vi "Pre-processing (White lines on ramp).vi"(6 "error in":errorcluster, 9 "Image In":T1) -> (0 "error out":errorcluster, 2 "Number of Particles":i32, 3 "Image Out":T1)   [LabVIEW 2009]
uses:
  <vilib>/vision/Image Controls.llb/IMAQ Image.ctl
  <vilib>/vision/NI_Vision_Development_Module.lvlib
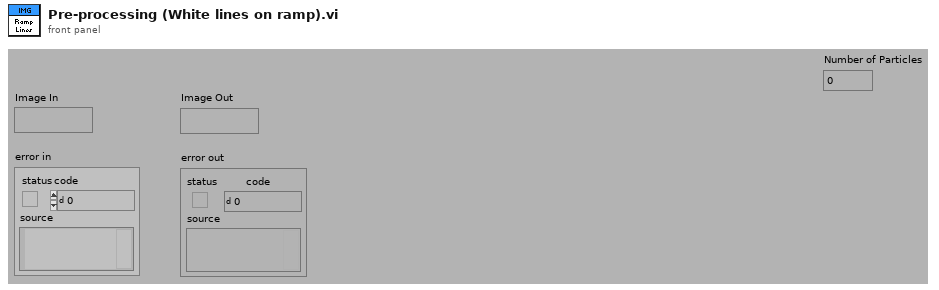
[diagram p1: front panel]
types:
  T1 = typedef "IMAQ Image.ctl" = refnum<image>
  T2 = cluster{"Measurement Parameter":i32, "Range Lower Value":dbl, "Range Upper Value":dbl, "Range":bool, "Measurement Type":bool}[]
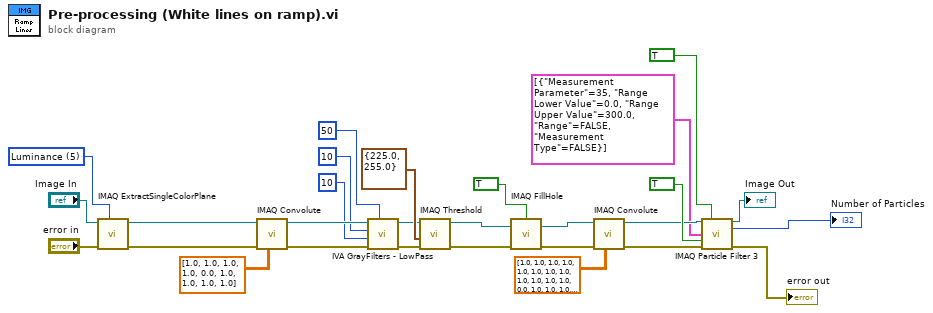
[diagram p0: block diagram]
diagram:
  w28 = 5 items=["Red", "Green", "Blue", "Hue", "Saturation", "Luminance", "Value", "Intensity"] ("Color Plane")
  n1 = call "IMAQ ExtractSingleColorPlane"("Color Plane"=w28, "error in (no error)"="error in", "Image Src"="Image In") -> ("error out"=w25:errorcluster, "Image Dst Out"=w23:T1)  [unwired: 1 in, 6 out]
  n2 = call "IMAQ Convolute"("Kernel"=sgl[][] [[1.0, 1.0, 1.0], [1.0, 0.0, 1.0], [1.0, 1.0, 1.0]], "error in (no error)"=w25, "Image Src"=w23) -> ("error out"=w22:errorcluster, "Image Dst Out"=w21:T1)  [unwired: 4 in, 3 out]
  n3 = call <vilib>:"IVA GrayFilters - LowPass.vi"("Tolerance"=50, "error in"=w22, "Filter size Y"=10, "Filter size X"=10, "Image In"=w21) -> ("error out"=w20:errorcluster, "Image Out"=w15:T1)  [unwired: 5 out]
  n4 = call "IMAQ Threshold"("error in (no error)"=w20, "Range"=cluster{"Lower value":sgl, "Upper value":sgl} {"Lower value"=225.0, "Upper value"=255.0}, "Image Src"=w15) -> ("error out"=w14:errorcluster, "Image Dst Out"=w12:T1)  [unwired: 3 in, 4 out]
  n5 = call "IMAQ FillHole"("error in (no error)"=w14, "Image Src"=w12, "Connectivity 4/8 (8)"=TRUE) -> ("error out"=w11:errorcluster, "Image Dst Out"=w9:T1)  [unwired: 1 in, 2 out]
  n6 = call "IMAQ Convolute"("Kernel"=sgl[][] [[1.0, 1.0, 1.0, 1.0, 1.0], [1.0, 1.0, 1.0, 1.0, 1.0], [1.0, 1.0, 0.0, 1.0, 1.0], [1.0, 1.0, 1.0, 1.0, 1.0], [1.0, 1.0, 1.0, 1.0, 1.0]], "error in (no error)"=w11, "Image Src"=w9) -> ("error out"=w8:errorcluster, "Image Dst Out"=w3:T1)  [unwired: 4 in, 3 out]
  n7 = call "IMAQ Particle Filter 3"("Image Src"=w3, "Connectivity 4/8 (8)"=TRUE, "Selection Values"=T2 [{"Measurement Parameter"=35, "Range Lower Value"=0.0, "Range Upper Value"=300.0, "Range"=FALSE, "Measurement Type"=FALSE}], "Keep/Remove Particles (F)"=TRUE ("Keep/Remove Particles"), "error in (no error)"=w8) -> ("Image Dst Out"=→"Image Out":T1, "Number of Particles"=→"Number of Particles":i32, "error out"=→"error out":errorcluster)  [unwired: 4 in, 4 out]
